vi "CCSDS Flatten.vi"(8 "error in (no error)":errorcluster, 9 "Packet Data in":string, 10 "Secondary Header in":string, 11 "CCSDS Primary Header in":T1 {"SeqFlags" format="%02b"; "Version" format="%03b"}) -> (0 "error out":errorcluster, 3 "CCSDS Packet out":string)   [LabVIEW 2018, in "TCPServer.lvlib"]
uses:
  TCPServer.lvlib
  TypeDefs/CCSDS.ctl
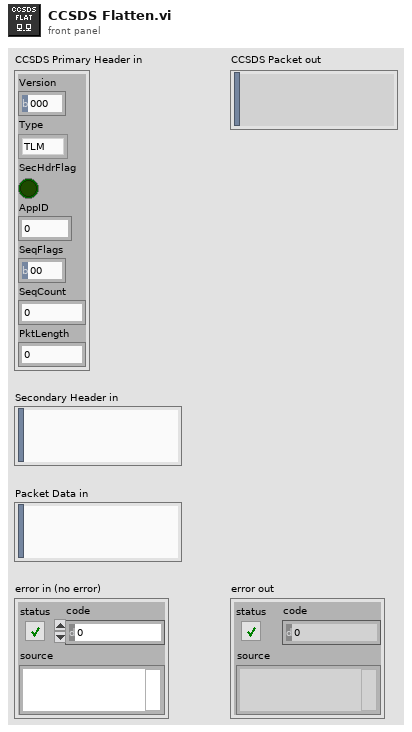
[diagram p1: front panel]
types:
  T1 = typedef "TCPServer.lvlib/CCSDS.ctl" = cluster{"Version":u8, "Type":enum8{"TLM", "CMD"}, "SecHdrFlag":bool, "AppID":u16, "SeqFlags":u8, "SeqCount":u16, "PktLength":u16}
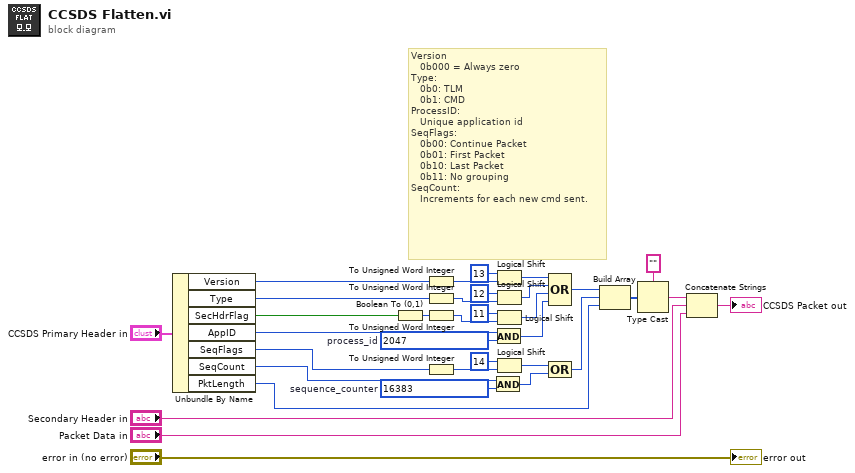
[diagram p0: block diagram]
diagram:
  w15 = u16 16383  # sequence_counter
  w22 = u16 2047  # process_id
  # "Version\n   0b000 = Always zero\nType:\n   0b0: TLM\n   0b1: CMD\nProcessID:\n   Unique application id\nSeqFlags:\n   0b00: Continue Packet\n   0b01: First Packet\n   0b10: Last Packet\n   0b11: No grouping\nSeqCount:\n   Increments for each new cmd sent."
  n1 = Unbundle By Name("CCSDS Primary Header in") -> ("Version"=w29:u8, "Type"=w26:enum8{"TLM", "CMD"}, "SecHdrFlag"=w28:bool, "AppID"=w21:u16, "SeqFlags"=w11:u8, "SeqCount"=w10:u16, "PktLength"=w14:u16)
  n2 = Boolean To (0,1)(Boolean=w28) -> (0, 1=w25:i16)
  n3 = To Unsigned Word Integer(number=w29) -> (unsigned 16bit integer=w27:u16)
  n4 = To Unsigned Word Integer(number=w26) -> (unsigned 16bit integer=w24:u16)
  n5 = To Unsigned Word Integer(number=w25) -> (unsigned 16bit integer=w23:u16)
  n6 = To Unsigned Word Integer(number=w11) -> (unsigned 16bit integer=w12:u16)
  n7 = And(x=w10, y=w15) -> (x .and. y?=w8:u16)
  n8 = Logical Shift(y=i16 13, x=w27) -> (x << y=w20:u16)
  n9 = Logical Shift(y=i16 12, x=w24) -> (x << y=w19:u16)
  n10 = Logical Shift(y=i16 11, x=w23) -> (x << y=w18:u16)
  n11 = And(x=w21, y=w22) -> (x .and. y?=w17:u16)
  n12 = Logical Shift(y=i16 14, x=w12) -> (x << y=w9:u16)
  n13 = Compound Arithmetic op=OR(w20, w19, w18, w17) -> (w16:u16)
  n14 = Compound Arithmetic op=OR(w9, w8) -> (w7:u16)
  n15 = Build Array(w16, w7, w14) -> (w34:u16[])
  n16 = Type Cast(type="", x=w34) -> (*(type *) &x=w5:string)
  n17 = Concatenate Strings(w5, "Secondary Header in", "Packet Data in") -> (→"CCSDS Packet out":string)
  "error out" <- "error in (no error)"
